vi "SATTdll.vi"(8 "error in (no error)":errorcluster, 11 "SAT Inputs":cluster{"t":dbl, "z":dbl[], "kph":u16}={"t"=313.15, "z"=[0.697614699375863, 0.302385300624138], "kph"=0} {"kph" items=["0", "1 = input x is liquid composition (bubble point)", "2 = input x is vapor composition (dew point)", "3 = input x is liquid composition (freezing point)", "4 = input x is vapor composition (sublimation point)"]}) -> (0 "error out":errorcluster, 3 "SAT Outputs":T1={"D"=nan, "e"=nan, "h"=nan, "p"=nan, "s"=nan, "t"=nan, "q"=nan, "Dl"=nan, "Dv"=nan, "x"=[nan, nan, 0.0, 0.0, 0.0, 0.0, 0.0, 0.0, 0.0, 0.0, 0.0, 0.0, 0.0, 0.0, 0.0, 0.0, 0.0, 0.0, 0.0, 0.0], "y"=[nan, nan, 0.0, 0.0, 0.0, 0.0, 0.0, 0.0, 0.0, 0.0, 0.0, 0.0, 0.0, 0.0, 0.0, 0.0, 0.0, 0.0, 0.0, 0.0], "nroot"=0, "k1"=0, "t1"=nan, "p1"=nan, "d1"=nan, "k2"=0, "t2"=nan, "p2"=nan, "d2"=nan, "k3"=0, "t3"=nan, "p3"=nan, "d3"=nan, "ierr"=0, "herr"="", "herr_length"=0})   [LabVIEW 2016]
doc: "subroutine SATTdll(t, z, kph, p, Dl, Dv, x, y, ierr, herr, herr_length)\n\nIterate for saturated liquid and vapor states given temperature\nand the composition of one phase\n\nINPUTS:\n t--temperature [K]\n if t is negative, then use other variables as\n initial guesses at abs(t)\n z--composition [array of mol frac] (phase specified by kph)\n kph--phase flag: 1 = input x is liquid composition (bubble point)\n 2 = input x is vapor composition (dew point)\n 3 = input x is liquid composition (freezing point)\n 4 = input x is vapor composition (sublimation point)\nOUTPUTS:\n p--pressure [kPa]\n Dl--molar density [mol/L] of saturated liquid\n Dv--molar density [mol/L] of saturated vapor\n For a pseudo pure fluid, the density of the equilibrium phase\n is not returned. Call SATT twice, once with kph=1 to get\n pliq and rhol, and once with kph=2 to get pvap and rhov.\n x--liquid phase composition [array of mol frac]\n y--vapor phase composition [array of mol frac]\n ierr--error flag: 0 = successful\n 1 = T < Tmin\n 8 = x out of range\n 9 = T and x out of range\n 120 = CRITP did not converge\n 121 = T > Tcrit\n 122 = TPRHO-liquid did not converge (pure fluid)\n 123 = TPRHO-vapor did not converge (pure fluid)\n 124 = pure fluid iteration did not converge\n following 3 error codes are advisory--iteration will either\n converge on later guess or error out (ierr = 128)\n -125 = TPRHO did not converge for parent ph (mix)\n -126 = TPRHO did not converge for incipient (mix)\n -127 = composition iteration did not converge\n 128 = mixture iteration did not converge\n herr--error string (character*255 variable if ierr<>0)\n herr_length -- length of variable herr (default: 255)"
uses:
  Ctl/SAT_Outputs.ctl
  REFPROP.DLL
panel:
  # "REFPROP-SATT_dll.vi"
  # "subroutine SATTdll(t, z, kph, p, dl, dv, x, y, ierr, herr, herr_length)"
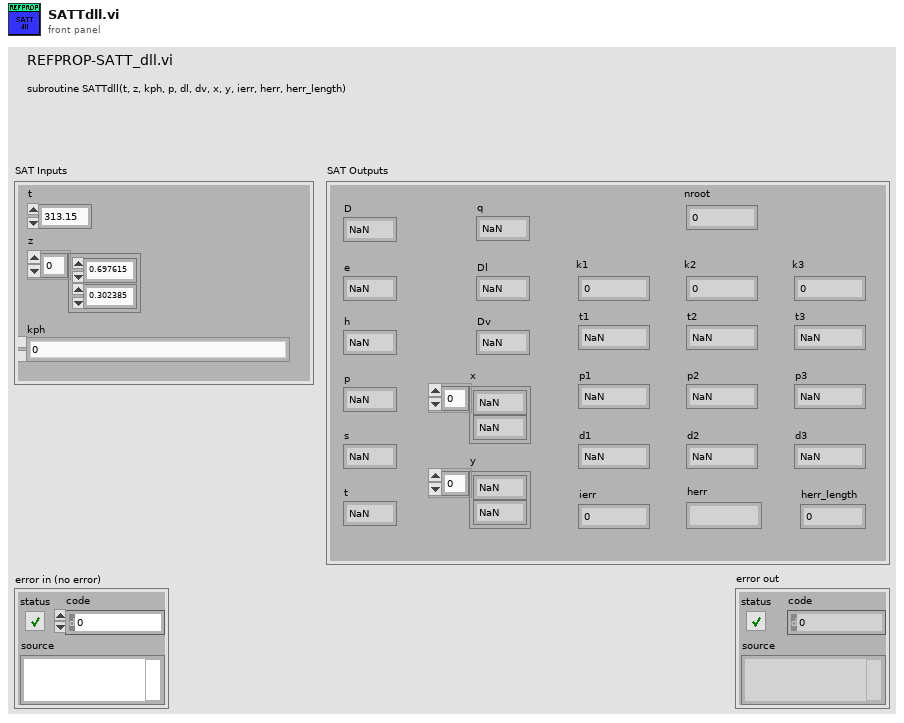
[diagram p1: front panel]
types:
  T1 = typedef "SAT_Outputs.ctl" = cluster{"D":dbl, "e":dbl, "h":dbl, "p":dbl, "s":dbl, "t":dbl, "q":dbl, "Dl":dbl, "Dv":dbl, "x":dbl[], "y":dbl[], "nroot":i32, "k1":i32, "t1":dbl, "p1":dbl, "d1":dbl, "k2":i32, "t2":dbl, "p2":dbl, "d2":dbl, "k3":i32, "t3":dbl, "p3":dbl, "d3":dbl, "ierr":i32, "herr":string, "herr_length":i32}
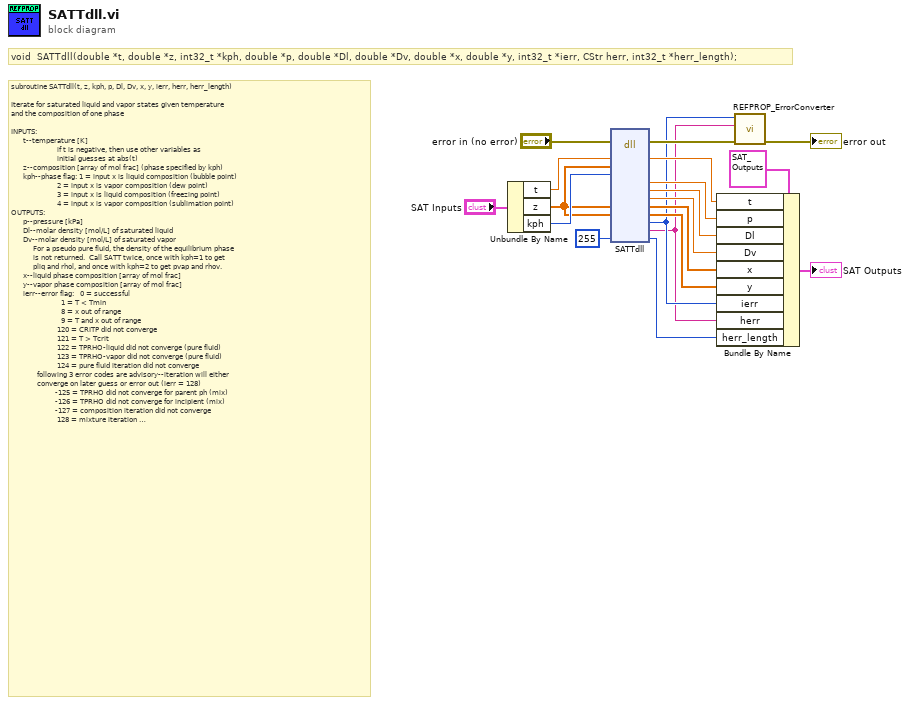
[diagram p0: block diagram]
diagram:
  # "void  SATTdll(double *t, double *z, int32_t *kph, double *p, double *Dl, double *Dv, double *x, double *y, int32_t *ierr, CStr herr, int32_t *herr_length);"
  # "subroutine SATTdll(t, z, kph, p, Dl, Dv, x, y, ierr, herr, herr_length)\n\nIterate for saturated liquid and vapor states given temperature\nand the composition of one phase\n\nINPUTS:\n      t--temperature [K]\n                       if t is negative, then use other variables as\n                       initial guesses at abs(t)\n      z--composition [array of mol frac] (phase specified by kph)\n      kph--phase flag: 1 = input x is liquid composition (bubble point)\n                       2 = input x is vapor composition (dew point)\n                       3 = input x is liquid composition (freezing point)\n                       4 = input x is vapor composition (sublimation point)\nOUTPUTS:\n      p--pressure [kPa]\n      Dl--molar density [mol/L] of saturated liquid\n      Dv--molar density [mol/L] of saturated vapor\n           For a pseudo pure fluid, the density of the equilibrium phase\n           is not returned.  Call SATT twice, once with kph=1 to get\n           pliq and rhol, and once with kph=2 to get pvap and rhov.\n      x--liquid phase composition [array of mol frac]\n      y--vapor phase composition [array of mol frac]\n      ierr--error flag:   0 = successful\n                         1 = T < Tmin\n                         8 = x out of range\n                         9 = T and x out of range\n                       120 = CRITP did not converge\n                       121 = T > Tcrit\n                       122 = TPRHO-liquid did not converge (pure fluid)\n                       123 = TPRHO-vapor did not converge (pure fluid)\n                       124 = pure fluid iteration did not converge\n             following 3 error codes are advisory--iteration will either\n             converge on later guess or error out (ierr = 128)\n                      -125 = TPRHO did not converge for parent ph (mix)\n                      -126 = TPRHO did not converge for incipient (mix)\n                      -127 = composition iteration did not converge\n                       128 = mixture iteration did not converge\n      herr--error string (character*255 variable if ierr<>0)\n      herr_length -- length of variable herr (default: 255)"
  n1 = Unbundle By Name("SAT Inputs") -> ("t"=w18:dbl, "z"=w12:dbl[], "kph"=w17:u16)
  n2 = dll-call lib="C:/Program Files (x86)/REFPROP/refprop.*" fn="SATTdll"(error in="error in (no error)", "t"=w18, "z"=w12, "kph"=w17, "x"=w12, "y"=w12, "herr_length"=255 ("ln")) -> (error out=w19:errorcluster, "t"=w9:dbl, "p"=w8:dbl, "Dl"=w7:dbl, "Dv"=w6:dbl, "x"=w5:dbl[], "y"=w4:dbl[], "ierr"=w3:i32, "herr"=w2:string, "herr_length"=w1:i32)  [unwired: 10 in, 1 out]
  n3 = Bundle By Name(cluster=T1 {"D"=nan, "e"=nan, "h"=nan, "p"=nan, "s"=nan, "t"=nan, "q"=0.0, "Dl"=nan, "Dv"=nan, "x"=[nan, nan, 0.0, 0.0, 0.0, 0.0, 0.0, 0.0, 0.0, 0.0, 0.0, 0.0, 0.0, 0.0, 0.0, 0.0, 0.0, 0.0, 0.0, 0.0], "y"=[nan, nan, 0.0, 0.0, 0.0, 0.0, 0.0, 0.0, 0.0, 0.0, 0.0, 0.0, 0.0, 0.0, 0.0, 0.0, 0.0, 0.0, 0.0, 0.0], "nroot"=0, "k1"=0, "t1"=nan, "p1"=nan, "d1"=nan, "k2"=0, "t2"=nan, "p2"=nan, "d2"=nan, "k3"=0, "t3"=nan, "p3"=nan, "d3"=nan, "ierr"=0, "herr"="", "herr_length"=0} ("SAT Outputs"), "t"=w9, "p"=w8, "Dl"=w7, "Dv"=w6, "x"=w5, "y"=w4, "ierr"=w3, "herr"=w2, "herr_length"=w1) -> (→"SAT Outputs":T1)
  n4 = call "REFPROP_ErrorConverter.vi"("error in (no error)"=w19, "Error Message"=w2, "Error Code"=w3) -> ("error out"=→"error out":errorcluster)  [unwired: 8 in]
